vi "Init.vi"(9 "Request":refnum<class "Request.lvclass">, 10 "Client":refnum<class "Client.lvclass">, 11 "OAuth2 in (New)":refnum<class "OAuth2.lvclass">) -> (3 "OAuth2":refnum<class "OAuth2.lvclass">)   [LabVIEW 2020, in "OAuth2.lvlib" / "OAuth2.lvclass"]
uses:
  OAuth2.lvclass
  Client/Client.lvclass
  Request/Request.lvclass
  OAuth2.lvclass/OAuth2.ctl
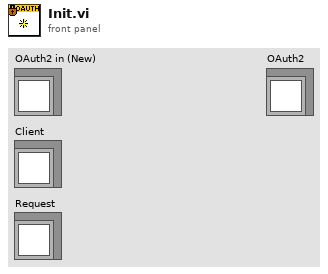
[diagram p1: front panel]
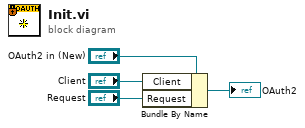
[diagram p0: block diagram]
diagram:
  n1 = Bundle By Name(cluster="OAuth2 in (New)", "Client"="Client", "Request"="Request") -> (→"OAuth2":refnum<class "OAuth2.lvclass">)
